vi "Stop_Main.vi"(1 "error in":errorcluster) -> (0 "error out":errorcluster)   [LabVIEW 2019]
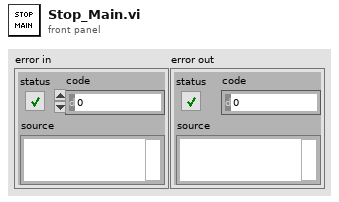
[diagram p1: front panel]
types:
  T1 = enum32{"Bad", "Idle", "Run top level", "Running"}
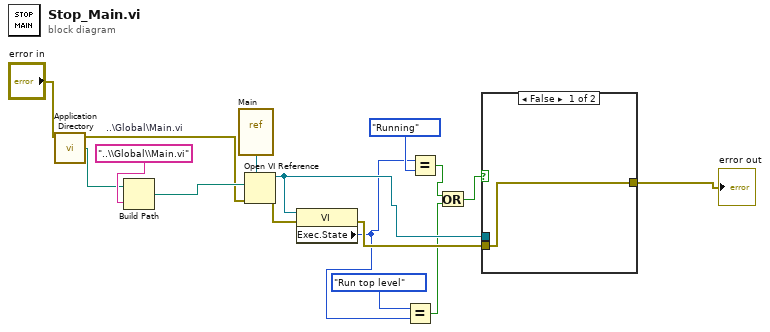
[diagram p0: block diagram]
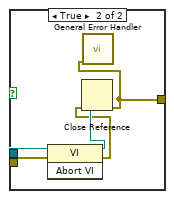
[diagram p2: hidden frame]
diagram:
  w14 = "..\\Global\\Main.vi"  # ..\Global\Main.vi
  n1 = call <vilib>:"Application Directory.vi"() -> ("Application Directory"=w13:path)
  n2 = Build Path(base path=w13, name or relative path=w14) -> (appended path=w12:path)
  n3 = vi-ref "Main.vi"() -> (w15:refnum<vi>)
  n4 = Open VI Reference ("VI-Referenz öffnen")(type specifier VI Refnum (for type only)=w15, vi path=w12, error in (no error)="error in") -> (vi reference=w11:refnum<vi>, error out=w10:errorcluster)  [unwired: 3 in]
  n5 = property class="VI"(reference=w11, error in=w10) -> (error out=w9:errorcluster, "Exec.State"=w4:T1)  [unwired: 1 out]
  n6 = Equal?(x=T1."Run top level" ("Execution:State"), y=w4) -> (x = y?=w3:bool)
  n7 = Equal?(x=w4, y=T1."Running" ("Execution:State")) -> (x = y?=w2:bool)
  n8 = Or(x=w2, y=w3) -> (x .or. y?=w1:bool)
  n9 = case shown="False" w1 {
    tunnel: w11 -> [_ w19]
    tunnel: w9 -> [w16 w18]
    tunnel: [w16 w17] -> w6
    frame False {
    }
    frame True {
      n10 = invoke class="VI" method="Abort VI"(reference=w19, error in=w18) -> (reference out=w21:refnum<vi>, error out=w20:errorcluster)  [unwired: 1 in, 1 out]
      n11 = Close Reference(reference=w21, error in (no error)=w20) -> (error out=w17:errorcluster)
      n12 = call <vilib>:"General Error Handler.vi"("error in (no error)"=w17) -> ()  [unwired: 10 in, 5 out]
    }
  }
  "error out" <- w6
